vi "Populate Attr XML Priv.vi"(0 "Attribute Names":string[](array[string]), 1 "Tab String":string, 2 "Data Types Dict":variant, 5 "Attribute Values":variant[](array[variant]), 12 "Include Type Attribute":bool=TRUE) -> (4 "Attr XML String":string)   [LabVIEW 2020, in "NI_VIAnCFGDataStructure.lvlib" / "Tree.lvclass"]
uses:
  <vilib>/addons/analyzer/VIAnCFGDataStructure/Tree Manager/Tree.lvclass
  <vilib>/addons/analyzer/VIAnCFGDataStructure/Tree Data/Tree Data.lvclass
  <vilib>/addons/analyzer/VIAnCFGDataStructure/Tree Manager/API/Generate Hash.vi
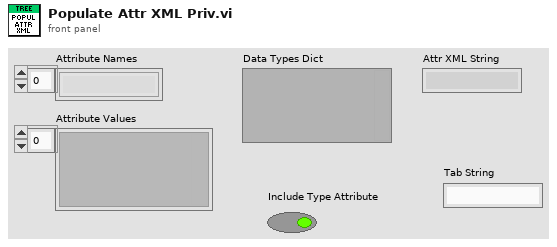
[diagram p1: front panel]
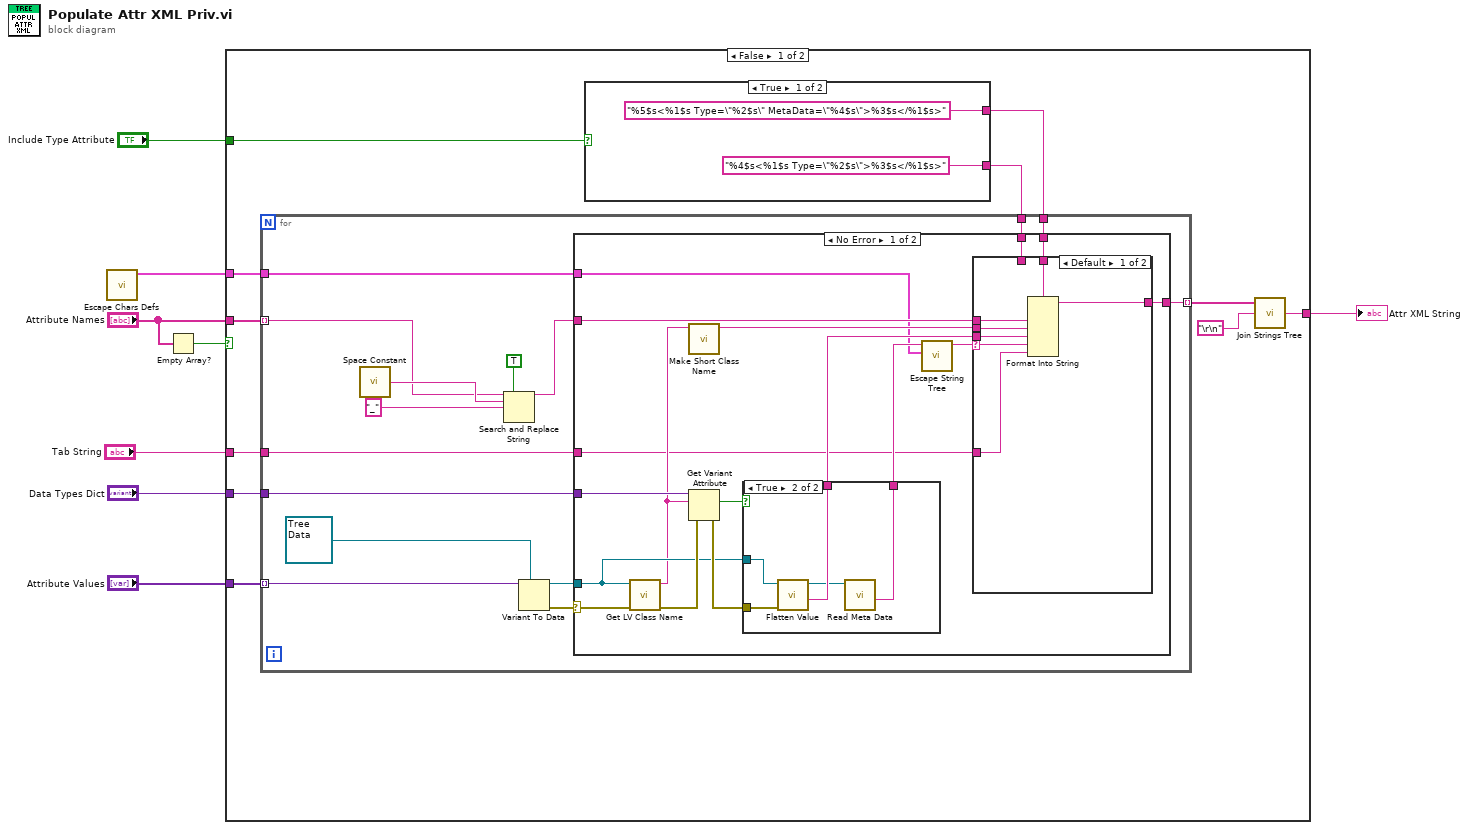
[diagram p0: block diagram]
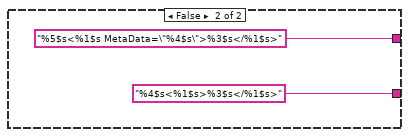
[diagram p2: hidden frame]
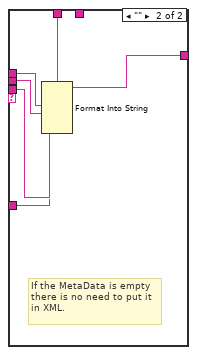
[diagram p3: hidden frame]
diagram:
  n1 = call <vilib>:"Escape Chars Defs.vi"() -> ("Escapes"=w6:cluster{"String":string, "Escape":string}[])  [unwired: 11 in]
  n2 = Empty Array?(array="Attribute Names") -> (empty?=w1:bool)
  n3 = case shown="False" w1 {
    tunnel: "Attribute Values" -> [w19 _]
    tunnel: "Data Types Dict" -> [w18 _]
    tunnel: w6 -> [w15 _]
    tunnel: "Include Type Attribute" -> [w14 _]
    tunnel: "Tab String" -> [w13 _]
    tunnel: [w12 _] -> w3
    tunnel: "Attribute Names" -> [w10 _]
    frame False {
      n4 = case shown="True" w14 {
        tunnel: ["%5$s<%1$s Type=\"%2$s\" MetaData=\"%4$s\">%3$s</%1$s>" ("format string") "%5$s<%1$s MetaData=\"%4$s\">%3$s</%1$s>" ("format string")] -> w17
        tunnel: ["%4$s<%1$s Type=\"%2$s\">%3$s</%1$s>" ("format string") "%4$s<%1$s>%3$s</%1$s>" ("format string")] -> w16
        frame True {
        }
        frame False {
        }
      }
      n5 = for {
        tunnel: w10 -> [w25] mode=indexing
        tunnel: w19 -> [w38] mode=indexing
        tunnel: w18 -> [w35]
        tunnel: w17 -> [w33]
        tunnel: w16 -> [w32]
        tunnel: [w31] -> w9 mode=indexing
        tunnel: w15 -> [w30]
        tunnel: w13 -> [w29]
        n6 = call <vilib>:"Space Constant.vi"() -> ("String"=w28:string)
        n7 = Search and Replace String(replace all?=TRUE ("replace all? (F)"), input string=w25, search string=w28, replace string="_") -> (result string=w24:string)  [unwired: 4 in, 3 out]
        n8 = Variant To Data(type=refnum<class "Tree Data.lvclass"> refnum ("Tree Data.lvclass"), Variant=w38) -> (data=w37:refnum<class "Tree Data.lvclass">, error out=w36:errorcluster)  [unwired: 1 in]
        n9 = case shown="No Error" w36 {
          selector: w36 -> [w55 _]
          tunnel: w37 -> [w50 _]
          tunnel: w24 -> [w49 _]
          tunnel: w35 -> [w54 _]
          tunnel: w33 -> [w48 _]
          tunnel: w32 -> [w46 _]
          tunnel: [w44 _] -> w31
          tunnel: w30 -> [w40 _]
          tunnel: w29 -> [w39 _]
          frame No Error {
            n10 = call <vilib>:"Get LV Class Name.vi"("error in (no error)"=w55, "object"=w50) -> ("error out"=w53:errorcluster, "class name"=w45:string)  [unwired: 8 in]
            n11 = call <vilib>:"Make Short Class Name.vi"("Class Name"=w45) -> ("Shortened Class Name"=w43:string)  [unwired: 10 in]
            n12 = Get Variant Attribute(Variant=w54, name=w45, error in=w53) -> (found=w51:bool, error out=w52:errorcluster)  [unwired: 1 in, 2 out]
            n13 = case shown="True" w51 {
              tunnel: [_ w73] -> w47
              tunnel: [_ w69] -> w42
              tunnel: w52 -> [_ w70]
              tunnel: w50 -> [_ w71]
              frame False {
              }
              frame True {
                n14 = call-dynamic "Flatten Value.vi"("Error In"=w70, "Tree Data In"=w71) -> ("Value"=w73:string, "Tree Data Out"=w72:refnum<class "Tree Data.lvclass">)  [unwired: 7 in, 1 out]
                n15 = call <vilib>:"Read Meta Data.vi"("Tree Data In"=w72) -> ("Meta Data"=w69:string)  [unwired: 9 in, 1 out]
              }
            }
            n16 = call <vilib>:"Escape String Tree.vi"("Escapes"=w40, "String In"=w42) -> ("String Out"=w41:string)  [unwired: 9 in]
            n17 = case shown="Default" w41 {
              selector: w41 -> [w58 _]
              tunnel: w43 -> [w60 w66]
              tunnel: w49 -> [w59 w67]
              tunnel: w48 -> [w62 _]
              tunnel: w47 -> [w61 w65]
              tunnel: w46 -> [_ w68]
              tunnel: [w57 w64] -> w44
              tunnel: w39 -> [w56 w63]
              frame Default {
                n18 = Format Into String(format string=w62, w59, w60, w61, w58, w56) -> (resulting string=w57:string)  [unwired: 2 in, 1 out]
              }
              frame "" {
                # "If the MetaData is empty\nthere is no need to put it\nin XML."
                n19 = Format Into String(format string=w68, w67, w66, w65, w63) -> (resulting string=w64:string)  [unwired: 2 in, 1 out]
              }
            }
          }
          frame Error {
          }
        }
      }
      n20 = call <vilib>:"Join Strings Tree.vi"("Separator (,)"="\r\n", "Strings In"=w9) -> ("String"=w12:string)  [unwired: 1 in]
    }
    frame True {
    }
  }
  "Attr XML String" <- w3
